vi "dbsys_login_init.vi"() -> (0 "Статус":i32, 1 "Вывод":string)   [LabVIEW 2017]
uses:
  DBSysCore.dll
panel:
  in  "Подтвердить":bool
  in  "coDecNumber":string
  in  "description":string
  in  "location":string
  in  "challengeTypeName":string
  in  "coParent":string
  in  "coVersion":string
  in  "coSerialNumber":string
  in  "coName":string
  in  "productName":string
  in  "Пароль":string
  in  "Логин":string
  # "Данные для авторизации в приложении\nпо обработке полученных результатов DBSysReport"
  # "Наименование изделия"
  # "Наименование объекта контроля"
  # "Серийный номер объекта контроля"
  # "Версия объекта контроля"
  # "Наименование внешнего модуля"
  # "Децимальный номер"
  # "Наименование типа испытания"
  # "Место проведения испытания"
  # "Описание"
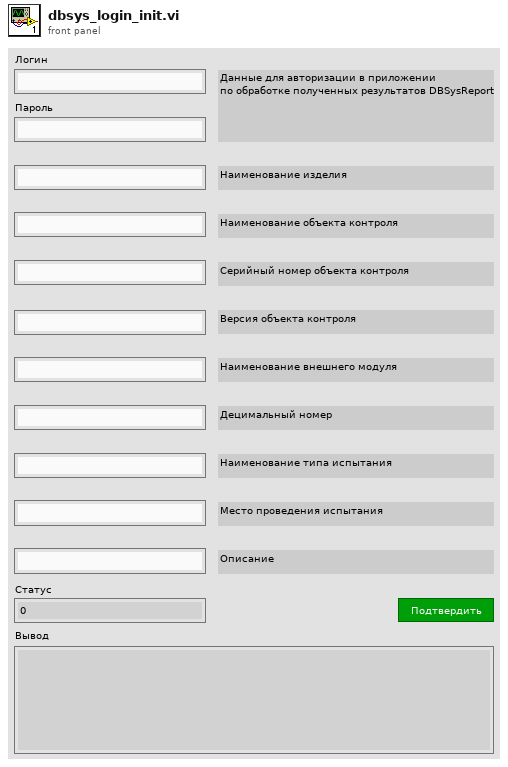
[diagram p1: front panel]
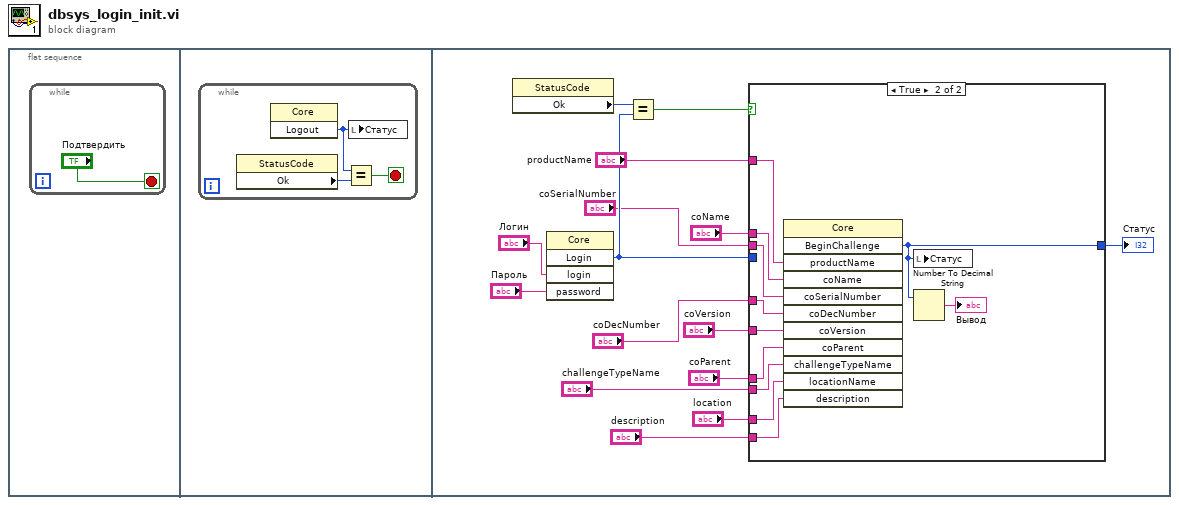
[diagram p0: block diagram]
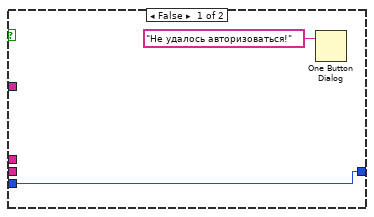
[diagram p2: hidden frame]
diagram:
  n1 = flat-sequence {
    frame #0 {
      n2 = while {
        stop <- "Подтвердить" stop-if-true
      }
    }
    frame #1 {
      n3 = while {
        stop <- w2 stop-if-true
        n4 = property class="StatusCode"() -> ("Ok"=w4:i32)  [unwired: 2 in, 2 out]
        n5 = invoke class="Core" method="Logout"() -> ("Logout"=w3:i32)  [unwired: 3 in, 2 out]
        n6 = Equal?(x=w3, y=w4) -> (x = y?=w2:bool)
        n7 = local write "Статус"(w3) -> ()
      }
    }
    frame #2 {
      n8 = property class="StatusCode"() -> ("Ok"=w5:i32)  [unwired: 2 in, 2 out]
      n9 = invoke class="Core" method="Login"("login"="Логин", "password"="Пароль") -> ("Login"=w18:i32)  [unwired: 3 in, 4 out]
      n10 = Equal?(x=w5, y=w18) -> (x = y?=w19:bool)
      n11 = case shown="True" w19 {
        tunnel: "coDecNumber" -> [_ w31]
        tunnel: "description" -> [_ w30]
        tunnel: "location" -> [_ w29]
        tunnel: "coVersion" -> [_ w28]
        tunnel: "coParent" -> [_ w27]
        tunnel: "coName" -> [_ w26]
        tunnel: "challengeTypeName" -> [_ w25]
        tunnel: "productName" -> [_ w24]
        tunnel: "coSerialNumber" -> [_ w23]
        tunnel: [w21 w22] -> w17
        tunnel: w18 -> [w21 _]
        frame False {
          n12 = One Button Dialog(message="Не удалось авторизоваться!") -> ()  [unwired: 1 in, 1 out]
        }
        frame True {
          n13 = invoke class="Core" method="BeginChallenge"("productName"=w24, "coName"=w26, "coSerialNumber"=w23, "coDecNumber"=w31, "coVersion"=w28, "coParent"=w27, "challengeTypeName"=w25, "locationName"=w29, "description"=w30) -> ("BeginChallenge"=w22:i32)  [unwired: 3 in, 11 out]
          n14 = local write "Статус"(w22) -> ()
          n15 = Number To Decimal String(number=w22) -> (decimal integer string=→"Вывод":string)  [unwired: 1 in]
        }
      }
      "Статус" <- w17
    }
  }
